vi "未命名 1.vi"() -> ()   [LabVIEW 2015]
uses:
  <vilib>/xnet/xnet.llb/XNET Frame CAN.ctl
  <vilib>/xnet/xnet.llb/XNET Frame Type CAN.ctl
  <vilib>/xnet/xnet.llb/XNET Create Session (Frame Output Single-point).vi
  <vilib>/xnet/xnet.llb/XNET Write (Frame CAN).vi
  <vilib>/xnet/xnet.llb/XNET Create Session (Frame Input Queued).vi
  <vilib>/xnet/xnet.llb/XNET Read (Frame CAN).vi
  <vilib>/xnet/xnet.llb/XNET Create Session (Frame Input Stream).vi
  <vilib>/xnet/xnet.llb/XNET Create Session (Frame Output Stream).vi
  <resource>/objmgr/xnet.rc
panel:
  out "PACK LEN":i32
  in  "data 3":T1[](array[typedef])=[{"timestamp"=timestamp(0 s since 1904-01-01), "payload"=[1, 2, 3, 4, 5, 6, 7, 8], "identifier"=2, "type"=0, "extended?"=FALSE, "echo?"=FALSE}, {"timestamp"=timestamp(0 s since 1904-01-01), "payload"=[0, 1, 2, 3, 4, 5, 6, 7], "identifier"=3, "type"=0, "extended?"=FALSE, "echo?"=FALSE}] {"payload" format="%x"; "timestamp" format="%<%.7X\n%x>T"; "type" items=["CAN Data"=0, "CAN Remote"=1, "CAN Bus Error"=2, "CAN 2.0 Data"=8, "CAN FD Data"=16, "CAN FD+BRS Data"=24, "J1939 Data"=192, "Delay"=224, "Log Trigger"=225, "Start Trigger"=226]; "identifier" format="%x"}
  in  "数组 2":refnum<k21>[](array[refnum])
  in  "stop":bool
  in  "Write":bool
  in  "Data Array":T1[](array[typedef]) {"payload" format="%x"; "timestamp" format="%<%.7X\n%x>T"; "type" items=["CAN Data"=0, "CAN Remote"=1, "CAN Bus Error"=2, "CAN 2.0 Data"=8, "CAN FD Data"=16, "CAN FD+BRS Data"=24, "J1939 Data"=192, "Delay"=224, "Log Trigger"=225, "Start Trigger"=226]; "identifier" format="%x"}
  in  "Select Interface 2":refnum<k21>="CAN1"
  out "Frames 2":string[][](table)
  in  "Number of Frames to Display 2":i32=15
  out "payload":u8[](array[numeric])
  out "Rec  ID":T1[](array[typedef]) {"payload" format="%x"; "timestamp" format="%<%.7X\n%x>T"; "type" items=["CAN Data"=0, "CAN Remote"=1, "CAN Bus Error"=2, "CAN 2.0 Data"=8, "CAN FD Data"=16, "CAN FD+BRS Data"=24, "J1939 Data"=192, "Delay"=224, "Log Trigger"=225, "Start Trigger"=226]; "identifier" format="%x"}
  out "identifier":u32
  out "Cluster":refnum<k21>
  out "数组":T1[](array[typedef]) {"payload" format="%x"; "timestamp" format="%<%.7X\n%x>T"; "type" items=["CAN Data"=0, "CAN Remote"=1, "CAN Bus Error"=2, "CAN 2.0 Data"=8, "CAN FD Data"=16, "CAN FD+BRS Data"=24, "J1939 Data"=192, "Delay"=224, "Log Trigger"=225, "Start Trigger"=226]; "identifier" format="%x"}
  out "Frames":string[][](table)
  in  "Hex Display":bool
  in  "Number of Frames to Display":i32=15
  in  "CAN frame":T1 {"payload" format="%x"; "timestamp" format="%<%.7X\n%x>T"; "type" items=["CAN Data"=0, "CAN Remote"=1, "CAN Bus Error"=2, "CAN 2.0 Data"=8, "CAN FD Data"=16, "CAN FD+BRS Data"=24, "J1939 Data"=192, "Delay"=224, "Log Trigger"=225, "Start Trigger"=226]; "identifier" format="%x"}
  in  "周期发送点火信号-显示端":T1[](array[typedef]) {"payload" format="%x"; "timestamp" format="%<%.7X\n%x>T"; "type" items=["CAN Data"=0, "CAN Remote"=1, "CAN Bus Error"=2, "CAN 2.0 Data"=8, "CAN FD Data"=16, "CAN FD+BRS Data"=24, "J1939 Data"=192, "Delay"=224, "Log Trigger"=225, "Start Trigger"=226]; "identifier" format="%x"}
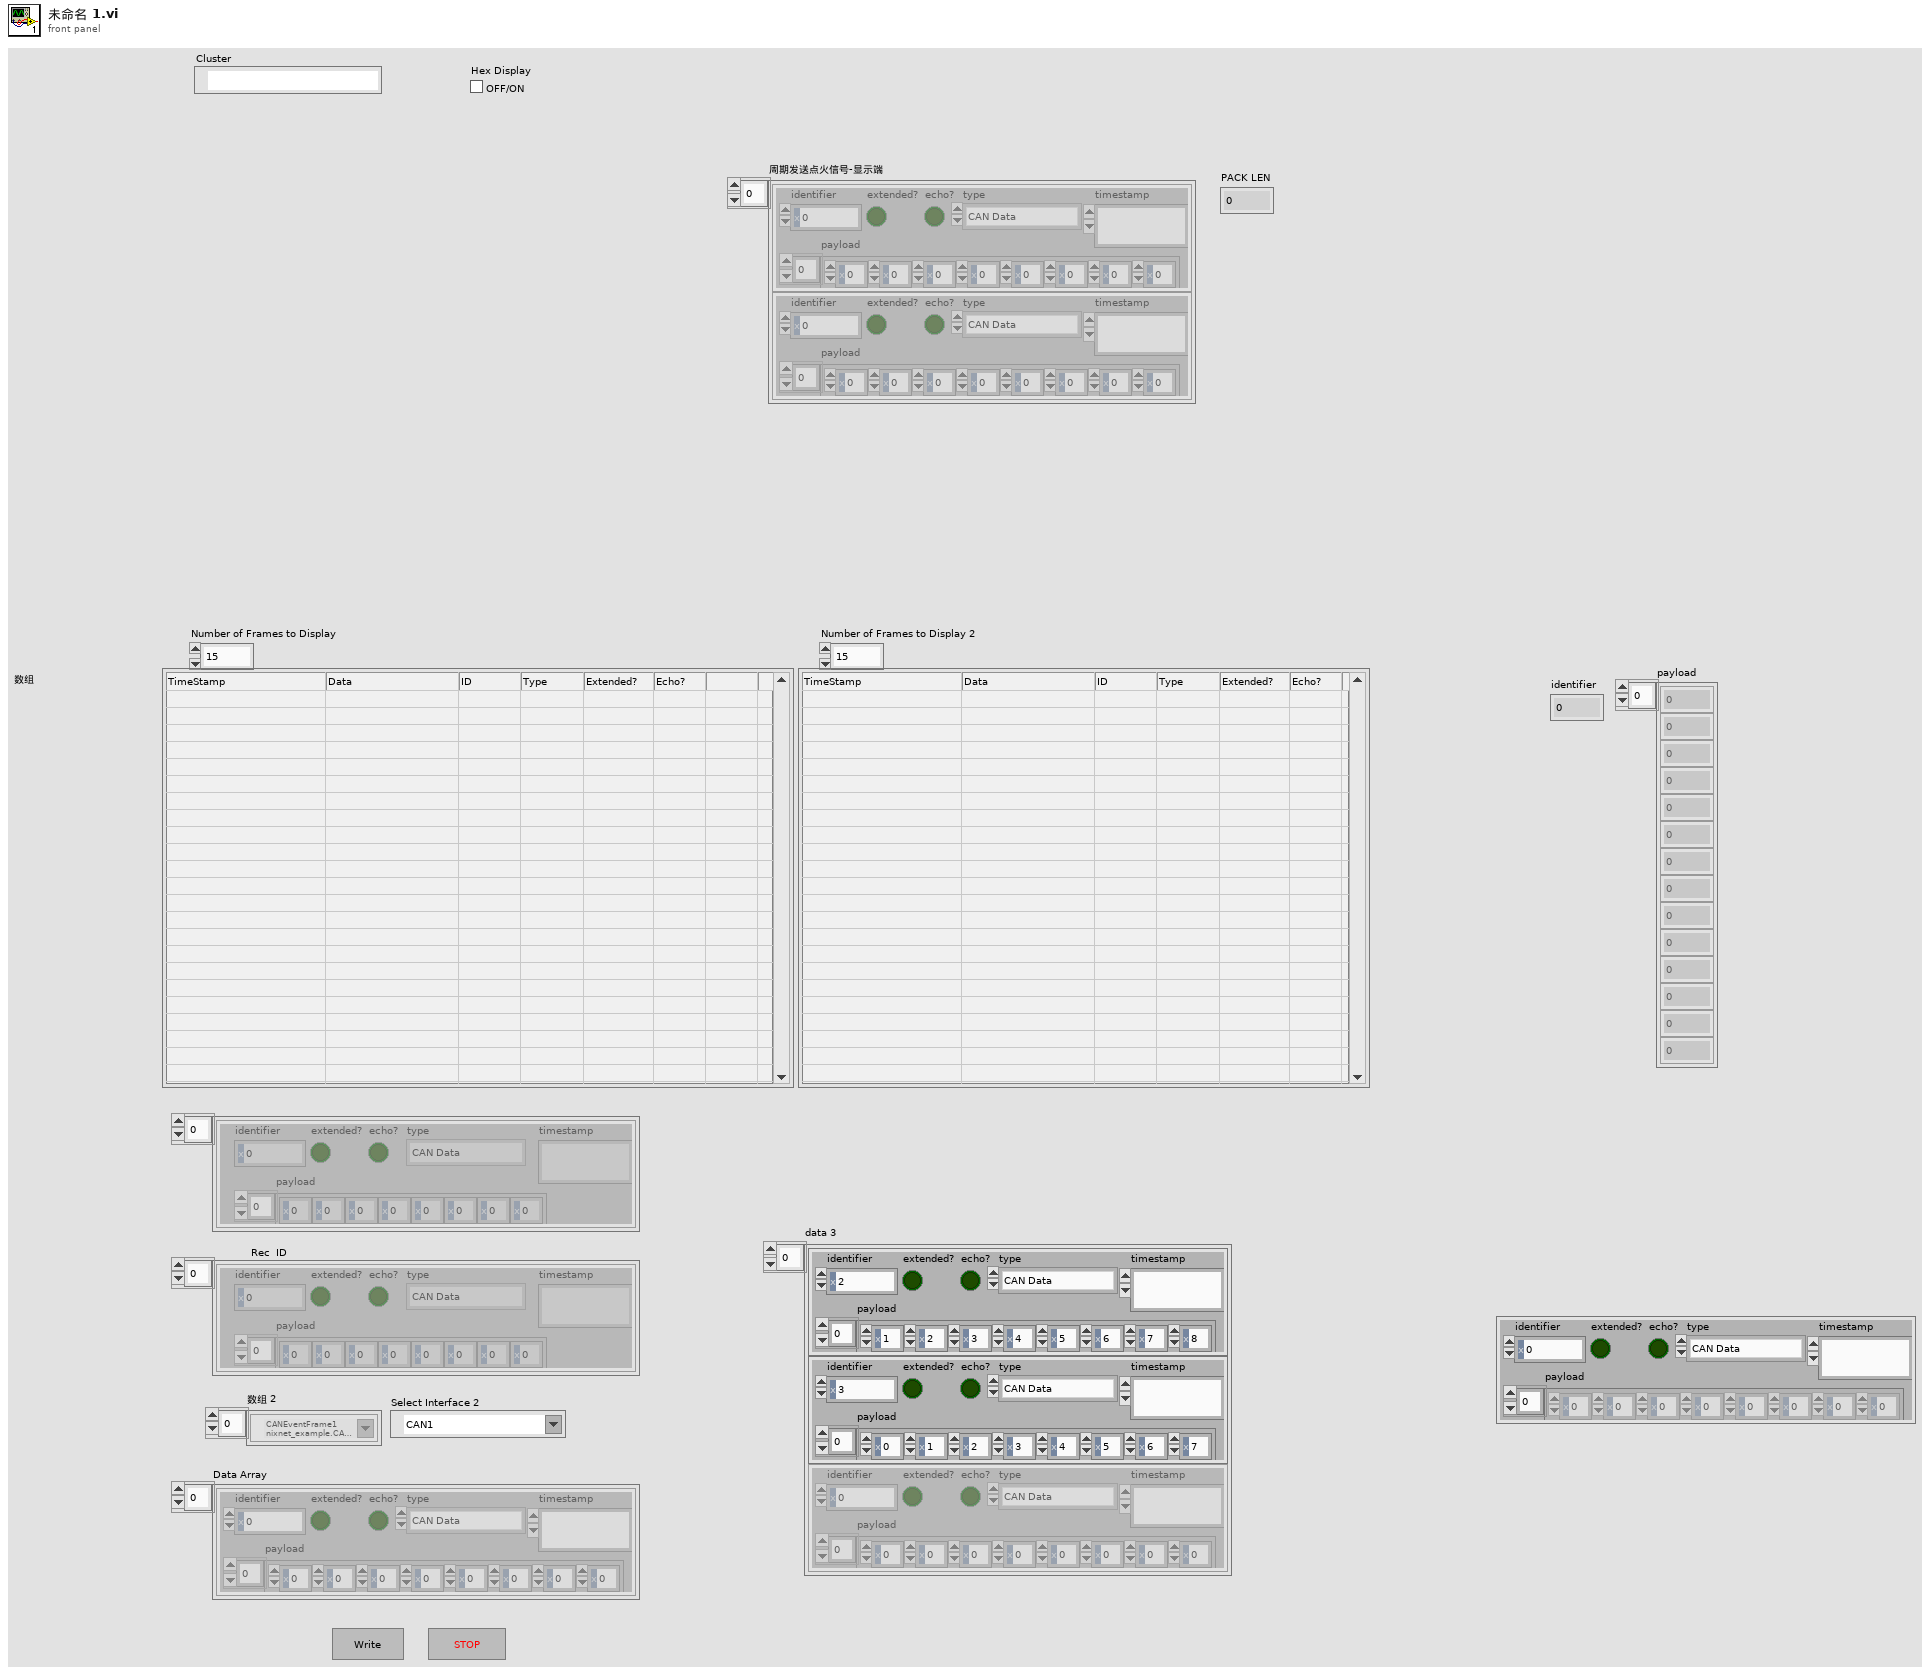
[diagram p1: front panel]
types:
  T1 = typedef "XNET Frame CAN.ctl" = cluster{"timestamp":timestamp, "payload":u8[], "identifier":u32, "type":T2, "extended?":bool, "echo?":bool}
  T2 = typedef "XNET Frame Type CAN.ctl" = u8
  T3 = cluster{"data[0]":T1, "data[1]":T1, "data[2]":T1, "data[3]":T1, "data[4]":T1, "data[5]":T1, "data[6]":T1, "data[7]":T1, "data[8]":T1}
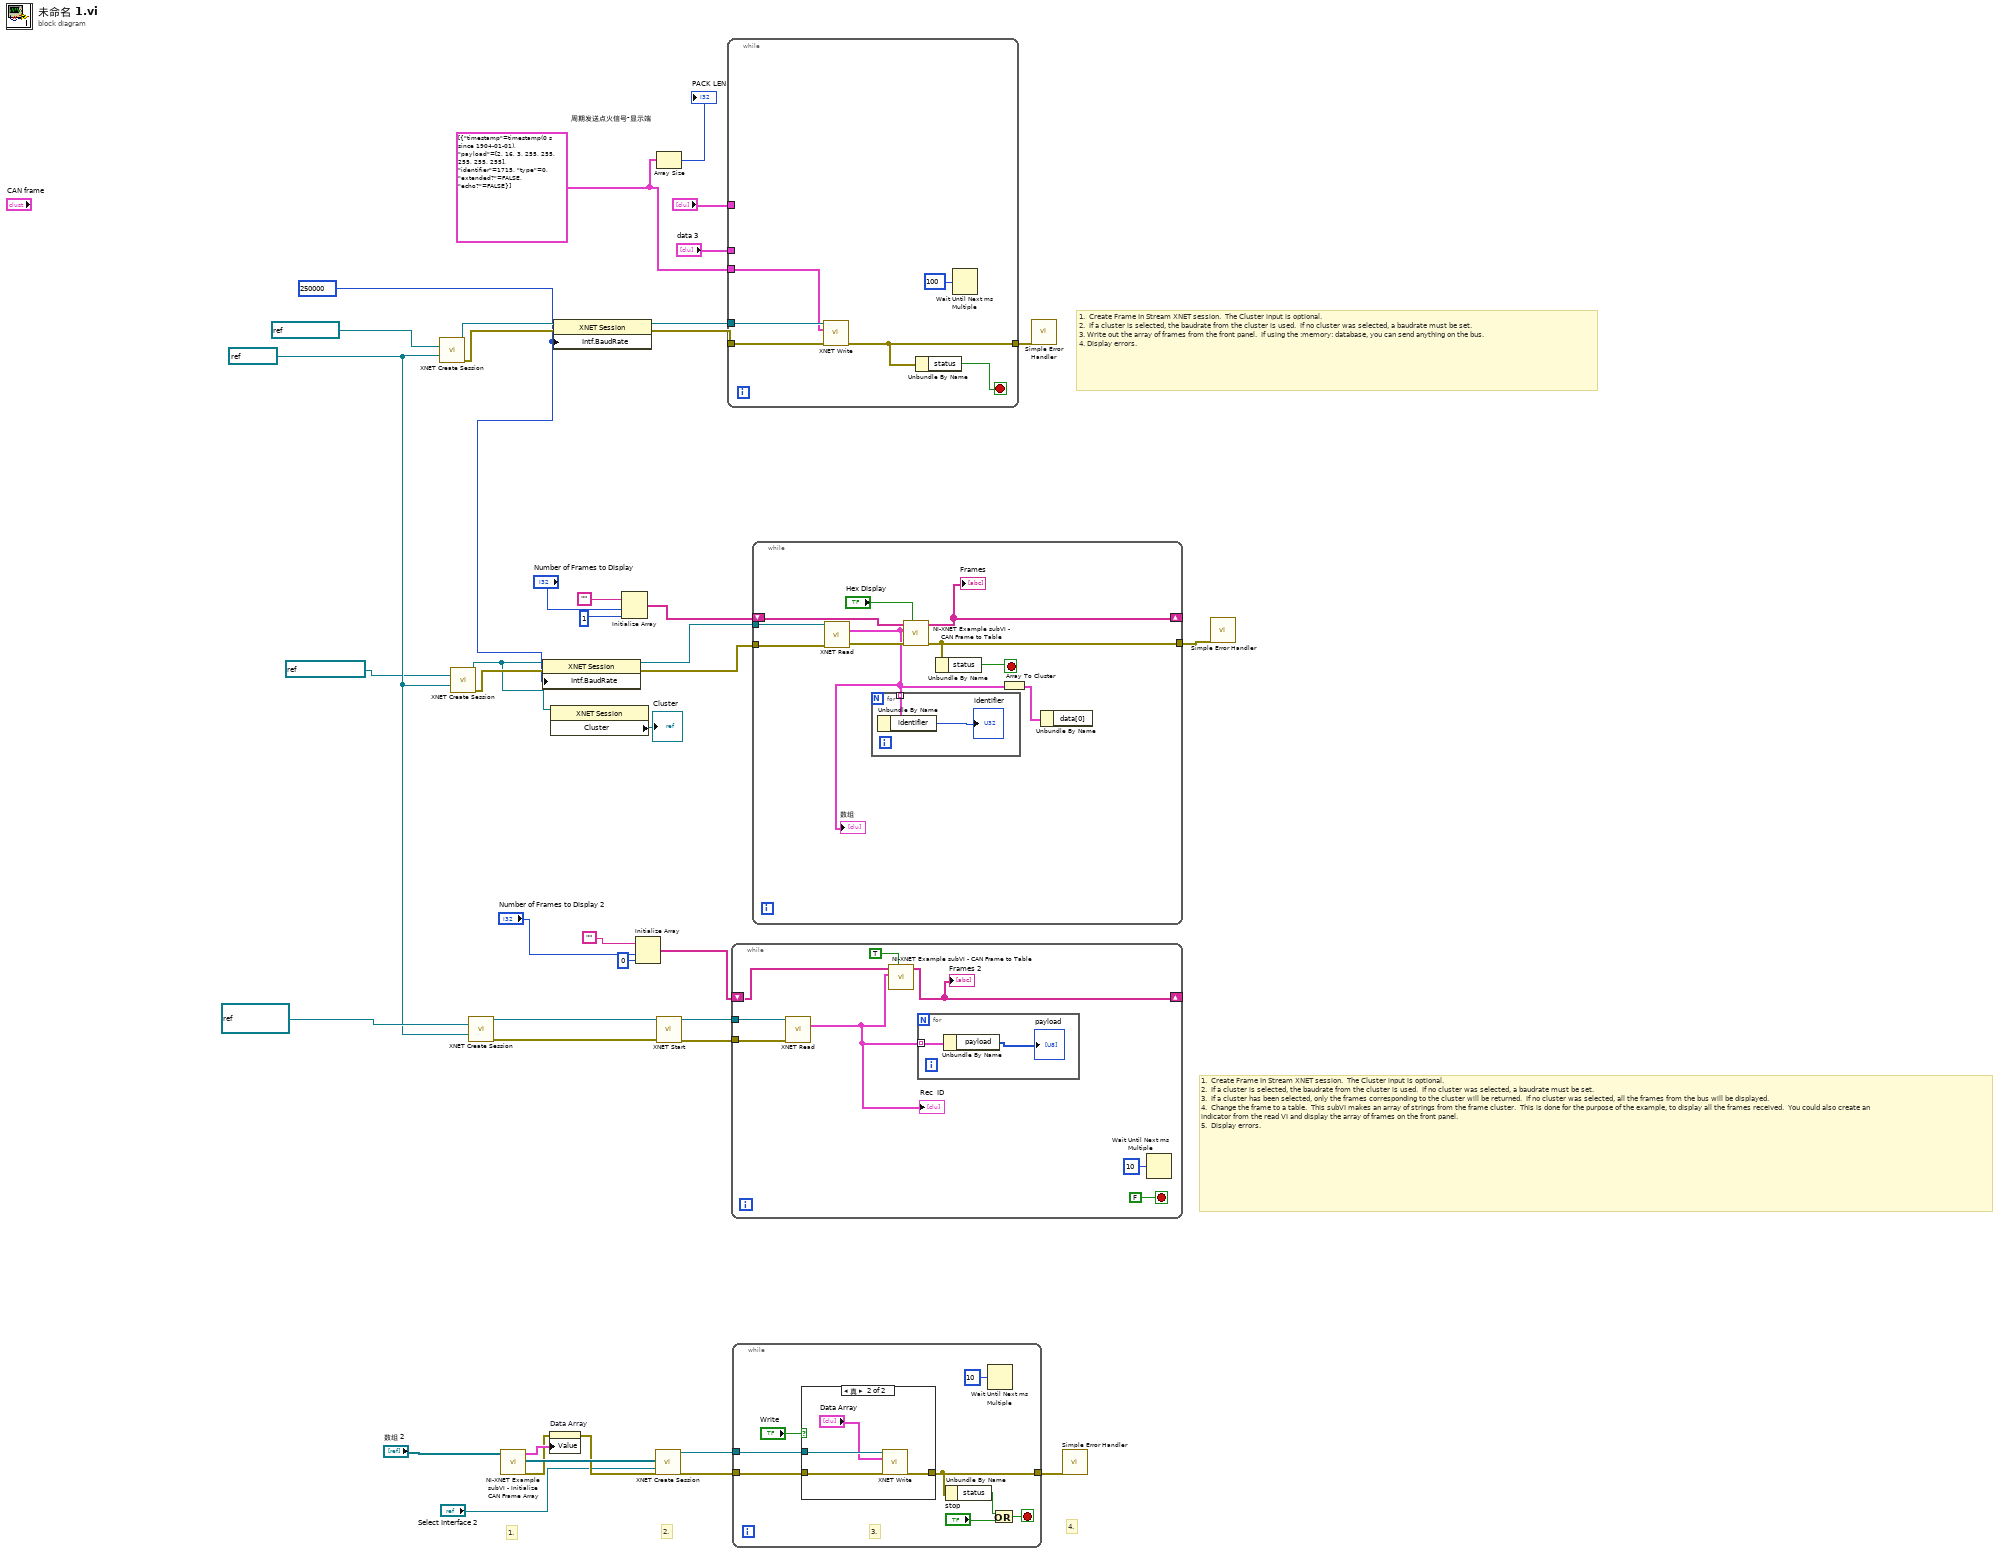
[diagram p0: block diagram]
diagram:
  w21 = refnum<k21> "CAN2" ("Select Interface")
  w28 = u32 250000 ("Interface Baud Rate")
  w2 = T1[] [{"timestamp"=timestamp(0 s since 1904-01-01), "payload"=[2, 16, 3, 255, 255, 255, 255, 255], "identifier"=1715, "type"=0, "extended?"=FALSE, "echo?"=FALSE}] ("Output Data")
  # "4."
  # "1."
  # "2."
  # "1.  Create Frame In Stream XNET session.  The Cluster input is optional.  \n2.  If a cluster is selected, the baudrate from the cluster is used.  If no cluster was selected, a baudrate must be set.\n3.  If a cluster has been selected, only the frames corresponding to the cluster will be returned.  If no cluster was selected, all the frames from the bus will be displayed.\n4.  Change the frame to a table.  This subVI makes an array of strings from the frame cluster.  This is done for the purpose of the example, to display all the frames received.  You could also create an indicator from the read VI and display the array of frames on the front panel. \n5.  Display errors."
  # "1.  Create Frame In Stream XNET session.  The Cluster input is optional.  \n2.  If a cluster is selected, the baudrate from the cluster is used.  If no cluster was selected, a baudrate must be set.\n3. Write out the array of frames from the front panel.  If using the :memory: database, you can send anything on the bus.\n4. Display errors."
  n1 = call-poly <vilib>:"XNET Create Session.vi"("cluster (:memory:)"=refnum<k21> "Z177TEST" ("CAN Cluster"), "interface"=w21) -> ("session out"=w41:refnum<k21>, "error out"=w38:errorcluster)  [unwired: 1 in, 11 out]
  n2 = call-poly <vilib>:"XNET Create Session.vi"("cluster (:memory:)"=refnum<k21> "Z177TEST" ("CAN Cluster"), "interface"=w21) -> ("session out"=w26:refnum<k21>, "error out"=w33:errorcluster)  [unwired: 1 in, 11 out]
  n3 = call-poly <vilib>:"XNET Create Session.vi"("frame"=refnum<k21> "Rec_59C\nZ177TEST", "interface"=w21) -> ("session out"=w24:refnum<k21>, "error out"=w20:errorcluster)  [unwired: 1 in, 11 out]
  n4 = call "NI-XNET Example subVI - Initialize CAN Frame Array.vi"("frame list in"="数组 2") -> ("error out"=w8:errorcluster, "frame list out"=w10:refnum<k21>[], "Data Array"=w9:T1[])  [unwired: 1 in, 5 out]
  n5 = property class="XNET Session"(reference=w26, error in=w33, "Intf.BaudRate"=w28) -> (reference out=w35:refnum<k21>, error out=w34:errorcluster)
  n6 = property on="Data Array" class="Arr (严格)"(error in=w8, "Value"=w9) -> (error out=w7:errorcluster)  [unwired: 1 in, 1 out]
  n7 = property class="XNET Session"(reference=w26) -> ("Cluster"=→"Cluster":refnum<k21>)  [unwired: 1 in, 2 out]
  n8 = property class="XNET Session"(reference=w41, error in=w38, "Intf.BaudRate"=w28) -> (reference out=w40:refnum<k21>, error out=w39:errorcluster)
  n9 = Initialize Array("", "Number of Frames to Display", 1 ("Dimension Size")) -> (w29:string[][])
  n10 = Initialize Array("", "Number of Frames to Display 2", 0 ("维数大小")) -> (w16:string[][])
  n11 = call-poly <vilib>:"XNET Create Session.vi"("frame list"=w10, "interface"="Select Interface 2", "error in (no error)"=w7) -> ("session out"=w12:refnum<k21>, "error out"=w11:errorcluster)  [unwired: 11 out]
  n12 = Array Size(array=w2) -> (size(s)=→"PACK LEN":i32)
  n13 = call <vilib>:"XNET Start.vi"("session in"=w24, "error in (no error)"=w20) -> ("session out"=w23:refnum<k21>, "error out"=w19:errorcluster)  [unwired: 12 in]
  n14 = while {
    tunnel: w40 -> [w47]
    tunnel: w39 -> [w46]
    tunnel: [w45] -> w37
    tunnel: "周期发送点火信号-显示端" -> [_]
    tunnel: "data 3" -> [_]
    tunnel: w2 -> [w42]
    stop <- w43 stop-if-true
    n15 = call-poly <vilib>:"XNET Write.vi"("session in"=w47, "data"=w42, "error in (no error)"=w46) -> ("error out"=w45:errorcluster)  [unwired: 12 out]
    n16 = Unbundle By Name(w45) -> ("status"=w43:bool)
    n17 = Wait Until Next ms Multiple(millisecond multiple=u32 100 ("milliseconds to wait")) -> ()  [unwired: 1 out]
  }
  n18 = while {
    tunnel: w23 -> [w55]
    tunnel: w19 -> [w53]
    shift-right: [w49] -> _
    shift-left: w16 -> [w51]
    stop <- FALSE stop-if-true
    n19 = call-poly <vilib>:"XNET Read.vi"("session in"=w55, "error in (no error)"=w53) -> ("data"=w50:T1[])  [unwired: 13 out]
    "Rec  ID" <- w50
    n20 = call "NI-XNET Example subVI - CAN Frame to Table.vi"("Hexadecimal?"=TRUE, "CAN Frames (from XNET Read)"=w50, "Input Array"=w51) -> ("Output Array"=w49:string[][])  [unwired: 2 in, 6 out]
    "Frames 2" <- w49
    n21 = for {
      tunnel: w50 -> [w57] mode=indexing
      n22 = Unbundle By Name(w57) -> ("payload"=→"payload":u8[])
    }
    n23 = Wait Until Next ms Multiple(millisecond multiple=u32 10 ("milliseconds to wait")) -> ()  [unwired: 1 out]
  }
  n24 = while {
    tunnel: w12 -> [w63]
    tunnel: w11 -> [w62]
    tunnel: [w61] -> w13
    stop <- w64 stop-if-true
    # "3."
    n25 = case shown="真" "Write" {
      tunnel: w63 -> [_ w70]
      tunnel: w62 -> [w66 w69]
      tunnel: [w66 w68] -> w61
      frame False {
      }
      frame True {
        n26 = call-poly <vilib>:"XNET Write.vi"("session in"=w70, "data"="Data Array", "error in (no error)"=w69) -> ("error out"=w68:errorcluster)  [unwired: 12 out]
      }
    }
    n27 = Unbundle By Name(w61) -> ("status"=w65:bool)
    n28 = Wait Until Next ms Multiple(millisecond multiple=u32 10 ("milliseconds to wait")) -> ()  [unwired: 1 out]
    n29 = Or(x=w65, y="stop") -> (x .or. y?=w64:bool)
  }
  n30 = while {
    tunnel: w35 -> [w80]
    tunnel: w34 -> [w79]
    tunnel: [w76] -> w36
    shift-right: [w73] -> _
    shift-left: w29 -> [w78]
    stop <- w74 stop-if-true
    n31 = call-poly <vilib>:"XNET Read.vi"("session in"=w80, "error in (no error)"=w79) -> ("data"=w71:T1[], "error out"=w77:errorcluster)  [unwired: 12 out]
    "数组" <- w71
    n32 = for {
      tunnel: w71 -> [w82] mode=indexing
      n33 = Unbundle By Name(w82) -> ("identifier"=→"identifier":u32)
    }
    n34 = call "NI-XNET Example subVI - CAN Frame to Table.vi"("Hexadecimal?"="Hex Display", "error in (no error)"=w77, "CAN Frames (from XNET Read)"=w71, "Input Array"=w78) -> ("error out"=w76:errorcluster, "Output Array"=w73:string[][])  [unwired: 1 in, 5 out]
    "Frames" <- w73
    n35 = Unbundle By Name(w76) -> ("status"=w74:bool)
    n36 = Array To Cluster(array=w71) -> (cluster=w72:T3)
    n37 = Unbundle By Name(w72) -> ()  [unwired: 1 out]
  }
  n38 = call <vilib>:"Simple Error Handler.vi"("error in (no error)"=w37) -> ()  [unwired: 1 in, 8 out]
  n39 = call <vilib>:"Simple Error Handler.vi"("error in (no error)"=w13) -> ()  [unwired: 1 in, 8 out]
  n40 = call <vilib>:"Simple Error Handler.vi"("error in (no error)"=w36) -> ()  [unwired: 1 in, 8 out]
